vi "Reset.vi"(11 "Hash Function in":refnum<class "NI_SHA-256.lvclass">) -> (3 "Hash Function out":refnum<class "NI_SHA-256.lvclass">)   [LabVIEW 2013, in "NI_SHA-256(2013).lvlib" / "NI_SHA-256.lvclass"]
uses:
  NI_SHA-256.lvclass
  NI_SHA-256.lvclass/NI_SHA-256.ctl
  subVIs/Mode.ctl
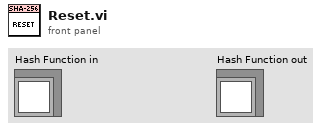
[diagram p1: front panel]
types:
  T1 = typedef "NI_SHA-256(2013).lvlib/NI_SHA-256.lvclass/Mode.ctl" = enum16{"SHA-256", "SHA-224"}
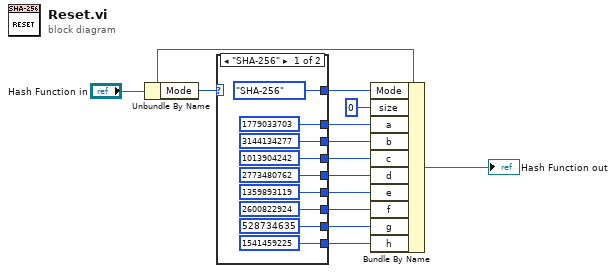
[diagram p0: block diagram]
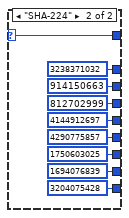
[diagram p2: hidden frame]
diagram:
  n1 = Unbundle By Name("Hash Function in") -> ("Mode"=w11:T1)
  n2 = case shown="\"SHA-256\"" w11 {
    selector: w11 -> [_ w23]
    tunnel: [u32 1779033703 ("Numeric") u32 3238371032 ("Numeric")] -> w9
    tunnel: [u32 3144134277 ("Numeric") u32 914150663 ("Numeric")] -> w8
    tunnel: [u32 1013904242 ("Numeric") u32 812702999 ("Numeric")] -> w7
    tunnel: [u32 2773480762 ("Numeric") u32 4144912697 ("Numeric")] -> w6
    tunnel: [u32 1359893119 ("Numeric") u32 4290775857 ("Numeric")] -> w5
    tunnel: [u32 2600822924 ("Numeric") u32 1750603025 ("Numeric")] -> w4
    tunnel: [u32 528734635 ("Numeric") u32 1694076839 ("Numeric")] -> w3
    tunnel: [u32 1541459225 ("Numeric") u32 3204075428 ("Numeric")] -> w2
    tunnel: [Mode."SHA-256" ("Mode") w23] -> w1
    frame "SHA-256" {
    }
    frame "SHA-224" {
    }
  }
  n3 = Bundle By Name(cluster="Hash Function in", "Mode"=w1, "size"=u64 0, "a"=w9, "b"=w8, "c"=w7, "d"=w6, "e"=w5, "f"=w4, "g"=w3, "h"=w2) -> (→"Hash Function out":refnum<class "NI_SHA-256.lvclass">)
